vi "Finish.vi"   [LabVIEW 2013]
doc: "This VI is called just before exiting. It is expected to close I/O refnum, save collected data, etc."
uses:
  <vilib>/Rock Robotics/WPI/Joystick/WPI_JoystickGetSetRefNum.vi
types:
  T1 = typedef "WPI_MotorControlDeviceRef.ctl" = cluster{"DeviceStatus":errorcluster, "Type":enum16{"PWM", "CAN"}, "PWM":cluster{"Digital Module":T2, "PWM Channel":T3, "DeadBand":T4}, "CAN":cluster{"Device Number":u8, "Control Mode":T5, "Semaphore":T6, "Max Vout":dbl}, "Invert":bool, "TransformRef":T7, "InvTransformRef":T7}
  T2 = typedef "FPGA_TypedefDigitalModule.ctl" = enum16{"Digital Module 1", "Digital Module 2"}
  T3 = typedef "FPGA_DIOPWMChannel.ctl" = enum8{"PWM 1", "PWM 2", "PWM 3", "PWM 4", "PWM 5", "PWM 6", "PWM 7", "PWM 8", "PWM 9", "PWM 10", "Invalid"}
  T4 = typedef "WPI_PWMDeadband.ctl" = cluster{"Name":string, "maxPositivePwm":i32, "minPositivePwm":i32, "centerPwm":i32, "maxNegativePwm":i32, "minNegativePwm":i32, "angularRange":u16}
  T5 = typedef "WPI_CANJaguar_ControlMode.ctl" = enum8{"Percent VBus", "Current", "Speed", "Position", "Voltage"}
  T6 = typedef "Semaphore RefNum" = refnum<k1>
  T7 = typedef "WPI_PWMTransform_ConPane.ctl" = refnum<vi>
  T8 = typedef "WPI_JoystickDevRef.ctl" = cluster{"Device":T9}
  T9 = typedef "WPI_JoystickDeviceEnum.ctl" = enum16{"USB 1", "USB 2", "USB 3", "USB 4", "Kinect 1", "Kinect 2"}
  T10 = typedef "WPI_CounterDevRef.ctl" = cluster{"DevStatus":errorcluster, "CntIndex":T11}
  T11 = typedef "FPGA_CounterCtrSystemIndex.ctl" = enum8{"Ctr 0", "Ctr 1", "Ctr 2", "Ctr 3", "Ctr 4", "Ctr 5", "Ctr 6", "Ctr 7", "Invalid"}
  T12 = typedef "WPI_SolenoidDevRef.ctl" = cluster{"DevStatus":errorcluster, "Solenoid Module":T13, "Forward Solenoid Channel":T14, "Reverse Solenoid Channel":T14}
  T13 = typedef "FPGA_TypedefSolenoidModule.ctl" = enum16{"Solenoid Module 1", "Solenoid Module 2"}
  T14 = typedef "WPI_SolenoidChannel.ctl" = enum8{"Solenoid 1", "Solenoid 2", "Solenoid 3", "Solenoid 4", "Solenoid 5", "Solenoid 6", "Solenoid 7", "Solenoid 8", "Invalid"}
  T15 = typedef "WPI_AnalogChannelDevRef.ctl" = cluster{"DevStatus":errorcluster, "Analog Module":T16, "Analog Channel":T17}
  T16 = typedef "FPGA_TypedefAnalogModule.ctl" = enum16{"Analog Module 1", "Analog Module 2"}
  T17 = typedef "FPGA_AIChannel.ctl" = enum8{"AI 1", "AI 2", "AI 3", "AI 4", "AI 5", "AI 6", "AI 7", "AI 8", "Invalid"}
  T18 = typedef "WPI_DigitalInputDevRef.ctl" = cluster{"DevStatus":errorcluster, "DIO Channel":T19, "Digital Module":T2}
  T19 = typedef "FPGA_DIOChannel.ctl" = enum8{"DIO 1", "DIO 2", "DIO 3", "DIO 4", "DIO 5", "DIO 6", "DIO 7", "DIO 8", "DIO 9", "DIO 10", "DIO 11", "DIO 12", "DIO 13", "DIO 14", "Invalid"}
  T20 = typedef "WPI_GyroDevRef.ctl" = cluster{"DevStatus":errorcluster, "Analog Module":T16, "Analog Channel":T17, "Offset":dbl, "Gain (VoltsPerDegree/Second)":dbl}
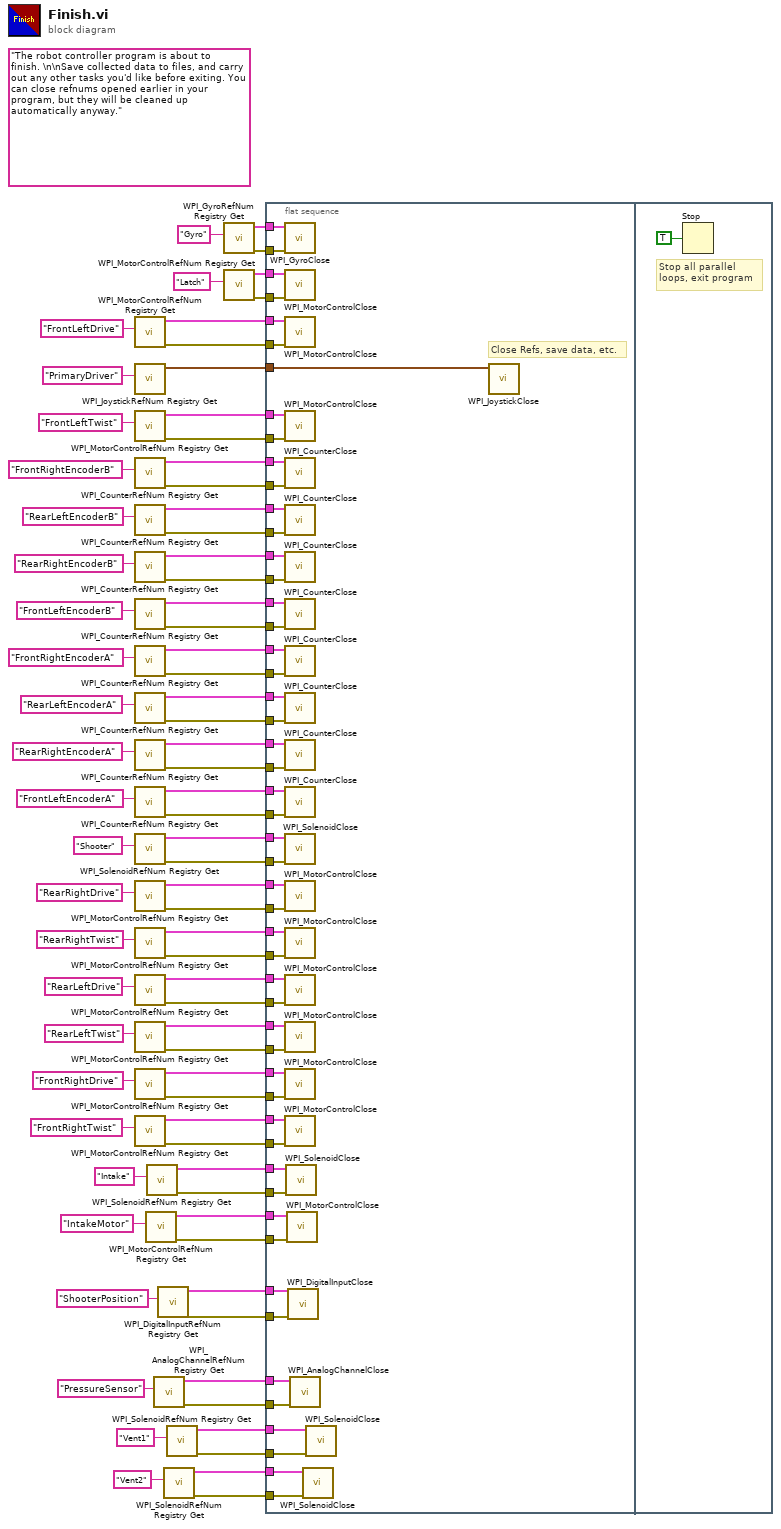
[diagram p0: block diagram]
diagram:
  (unwired) "The robot controller program is about to finish. \n\nSave collected data to files, and carry out any other tasks you'd like before exiting. You can close refnums opened earlier in your program, but they will be cleaned up automatically anyway."
  n1 = call <vilib>:"WPI_MotorControlRefNum Registry Get.vi"("refnum name"="FrontLeftDrive") -> ("error out"=w70:errorcluster, "MotorControlDevRef"=w71:T1)  [unwired: 9 in]
  n2 = call <vilib>:"WPI_JoystickRefNum Registry Get.vi"("refnum name"="PrimaryDriver") -> ("JoystickDevRef"=w77:T8)  [unwired: 9 in, 1 out]
  n3 = call <vilib>:"WPI_MotorControlRefNum Registry Get.vi"("refnum name"="FrontLeftTwist") -> ("error out"=w74:errorcluster, "MotorControlDevRef"=w75:T1)  [unwired: 9 in]
  n4 = call <vilib>:"WPI_CounterRefNum Registry Get.vi"("refnum name"="FrontRightEncoderB") -> ("error out"=w30:errorcluster, "CounterDevRef"=w29:T10)  [unwired: 9 in]
  n5 = call <vilib>:"WPI_CounterRefNum Registry Get.vi"("refnum name"="RearLeftEncoderB") -> ("error out"=w31:errorcluster, "CounterDevRef"=w28:T10)  [unwired: 9 in]
  n6 = call <vilib>:"WPI_CounterRefNum Registry Get.vi"("refnum name"="RearRightEncoderB") -> ("error out"=w32:errorcluster, "CounterDevRef"=w27:T10)  [unwired: 9 in]
  n7 = call <vilib>:"WPI_CounterRefNum Registry Get.vi"("refnum name"="FrontLeftEncoderB") -> ("error out"=w33:errorcluster, "CounterDevRef"=w26:T10)  [unwired: 9 in]
  n8 = call <vilib>:"WPI_CounterRefNum Registry Get.vi"("refnum name"="FrontRightEncoderA") -> ("error out"=w37:errorcluster, "CounterDevRef"=w38:T10)  [unwired: 9 in]
  n9 = call <vilib>:"WPI_CounterRefNum Registry Get.vi"("refnum name"="RearLeftEncoderA") -> ("error out"=w36:errorcluster, "CounterDevRef"=w39:T10)  [unwired: 9 in]
  n10 = call <vilib>:"WPI_CounterRefNum Registry Get.vi"("refnum name"="RearRightEncoderA") -> ("error out"=w35:errorcluster, "CounterDevRef"=w40:T10)  [unwired: 9 in]
  n11 = call <vilib>:"WPI_CounterRefNum Registry Get.vi"("refnum name"="FrontLeftEncoderA") -> ("error out"=w34:errorcluster, "CounterDevRef"=w41:T10)  [unwired: 9 in]
  n12 = call <vilib>:"WPI_SolenoidRefNum Registry Get.vi"("refnum name"="Shooter") -> ("error out"=w47:errorcluster, "SolenoidDevRef"=w48:T12)  [unwired: 9 in]
  n13 = call <vilib>:"WPI_MotorControlRefNum Registry Get.vi"("refnum name"="RearRightDrive") -> ("error out"=w57:errorcluster, "MotorControlDevRef"=w56:T1)  [unwired: 9 in]
  n14 = call <vilib>:"WPI_MotorControlRefNum Registry Get.vi"("refnum name"="RearRightTwist") -> ("error out"=w55:errorcluster, "MotorControlDevRef"=w54:T1)  [unwired: 9 in]
  n15 = call <vilib>:"WPI_MotorControlRefNum Registry Get.vi"("refnum name"="RearLeftDrive") -> ("error out"=w58:errorcluster, "MotorControlDevRef"=w59:T1)  [unwired: 9 in]
  n16 = call <vilib>:"WPI_MotorControlRefNum Registry Get.vi"("refnum name"="RearLeftTwist") -> ("error out"=w60:errorcluster, "MotorControlDevRef"=w61:T1)  [unwired: 9 in]
  n17 = call <vilib>:"WPI_MotorControlRefNum Registry Get.vi"("refnum name"="FrontRightDrive") -> ("error out"=w64:errorcluster, "MotorControlDevRef"=w65:T1)  [unwired: 9 in]
  n18 = call <vilib>:"WPI_MotorControlRefNum Registry Get.vi"("refnum name"="FrontRightTwist") -> ("error out"=w66:errorcluster, "MotorControlDevRef"=w67:T1)  [unwired: 9 in]
  n19 = call <vilib>:"WPI_MotorControlRefNum Registry Get.vi"("refnum name"="IntakeMotor") -> ("error out"=w18:errorcluster, "MotorControlDevRef"=w17:T1)  [unwired: 9 in]
  n20 = call <vilib>:"WPI_SolenoidRefNum Registry Get.vi"("refnum name"="Intake") -> ("error out"=w14:errorcluster, "SolenoidDevRef"=w13:T12)  [unwired: 9 in]
  n21 = call <vilib>:"WPI_AnalogChannelRefNum Registry Get.vi"("refnum name"="PressureSensor") -> ("error out"=w8:errorcluster, "AIDeviceRef"=w9:T15)  [unwired: 9 in]
  n22 = call <vilib>:"WPI_DigitalInputRefNum Registry Get.vi"("refnum name"="ShooterPosition") -> ("error out"=w11:errorcluster, "DigitalInputDevRef"=w12:T18)  [unwired: 9 in]
  n23 = call <vilib>:"WPI_SolenoidRefNum Registry Get.vi"("refnum name"="Vent2") -> ("error out"=w2:errorcluster, "SolenoidDevRef"=w1:T12)  [unwired: 9 in]
  n24 = call <vilib>:"WPI_SolenoidRefNum Registry Get.vi"("refnum name"="Vent1") -> ("error out"=w5:errorcluster, "SolenoidDevRef"=w6:T12)  [unwired: 9 in]
  n25 = call <vilib>:"WPI_GyroRefNum Registry Get.vi"("refnum name"="Gyro") -> ("error out"=w20:errorcluster, "GyroDevRef"=w21:T20)  [unwired: 9 in]
  n26 = call <vilib>:"WPI_MotorControlRefNum Registry Get.vi"("refnum name"="Latch") -> ("error out"=w49:errorcluster, "MotorControlDevRef"=w50:T1)  [unwired: 9 in]
  n27 = flat-sequence {
    tunnel: w77 -> [w128]
    tunnel: w75 -> [w127]
    tunnel: w74 -> [w126]
    tunnel: w71 -> [w124]
    tunnel: w70 -> [w125]
    tunnel: w67 -> [w123]
    tunnel: w66 -> [w122]
    tunnel: w65 -> [w121]
    tunnel: w64 -> [w120]
    tunnel: w61 -> [w119]
    tunnel: w60 -> [w118]
    tunnel: w59 -> [w117]
    tunnel: w58 -> [w116]
    tunnel: w54 -> [w112]
    tunnel: w55 -> [w113]
    tunnel: w56 -> [w114]
    tunnel: w57 -> [w115]
    tunnel: w50 -> [w111]
    tunnel: w49 -> [w110]
    tunnel: w48 -> [w109]
    tunnel: w47 -> [w108]
    tunnel: w41 -> [w107]
    tunnel: w40 -> [w106]
    tunnel: w39 -> [w105]
    tunnel: w38 -> [w104]
    tunnel: w37 -> [w103]
    tunnel: w36 -> [w102]
    tunnel: w35 -> [w101]
    tunnel: w34 -> [w100]
    tunnel: w26 -> [w92]
    tunnel: w27 -> [w93]
    tunnel: w28 -> [w94]
    tunnel: w29 -> [w95]
    tunnel: w30 -> [w96]
    tunnel: w31 -> [w97]
    tunnel: w32 -> [w98]
    tunnel: w33 -> [w99]
    tunnel: w21 -> [w91]
    tunnel: w20 -> [w90]
    tunnel: w17 -> [w88]
    tunnel: w18 -> [w89]
    tunnel: w13 -> [w86]
    tunnel: w14 -> [w87]
    tunnel: w12 -> [w85]
    tunnel: w11 -> [w84]
    tunnel: w9 -> [w83]
    tunnel: w8 -> [w82]
    tunnel: w6 -> [w81]
    tunnel: w5 -> [w80]
    tunnel: w1 -> [w78]
    tunnel: w2 -> [w79]
    frame #0 {
      # "Close Refs, save data, etc."
      n28 = call <vilib>:"WPI_GyroClose.vi"("error in (no error)"=w90, "GyroDevRef"=w91) -> ()  [unwired: 9 in, 1 out]
      n29 = call <vilib>:"WPI_MotorControlClose.vi"("error in (no error)"=w110, "MotorControlDevRef"=w111) -> ()  [unwired: 9 in, 1 out]
      n30 = call <vilib>:"WPI_MotorControlClose.vi"("error in (no error)"=w125, "MotorControlDevRef"=w124) -> ()  [unwired: 9 in, 1 out]
      n31 = call <vilib>:"WPI_MotorControlClose.vi"("error in (no error)"=w126, "MotorControlDevRef"=w127) -> ()  [unwired: 9 in, 1 out]
      n32 = call <vilib>:"WPI_CounterClose.vi"("error in (no error)"=w96, "CounterDevRef"=w95) -> ()  [unwired: 9 in, 1 out]
      n33 = call <vilib>:"WPI_CounterClose.vi"("error in (no error)"=w97, "CounterDevRef"=w94) -> ()  [unwired: 9 in, 1 out]
      n34 = call <vilib>:"WPI_CounterClose.vi"("error in (no error)"=w98, "CounterDevRef"=w93) -> ()  [unwired: 9 in, 1 out]
      n35 = call <vilib>:"WPI_CounterClose.vi"("error in (no error)"=w99, "CounterDevRef"=w92) -> ()  [unwired: 9 in, 1 out]
      n36 = call <vilib>:"WPI_CounterClose.vi"("error in (no error)"=w103, "CounterDevRef"=w104) -> ()  [unwired: 9 in, 1 out]
      n37 = call <vilib>:"WPI_CounterClose.vi"("error in (no error)"=w102, "CounterDevRef"=w105) -> ()  [unwired: 9 in, 1 out]
      n38 = call <vilib>:"WPI_CounterClose.vi"("error in (no error)"=w101, "CounterDevRef"=w106) -> ()  [unwired: 9 in, 1 out]
      n39 = call <vilib>:"WPI_CounterClose.vi"("error in (no error)"=w100, "CounterDevRef"=w107) -> ()  [unwired: 9 in, 1 out]
      n40 = call <vilib>:"WPI_SolenoidClose.vi"("error in (no error)"=w108, "SolenoidDevRef"=w109) -> ()  [unwired: 9 in, 1 out]
      n41 = call <vilib>:"WPI_MotorControlClose.vi"("error in (no error)"=w115, "MotorControlDevRef"=w114) -> ()  [unwired: 9 in, 1 out]
      n42 = call <vilib>:"WPI_MotorControlClose.vi"("error in (no error)"=w113, "MotorControlDevRef"=w112) -> ()  [unwired: 9 in, 1 out]
      n43 = call <vilib>:"WPI_MotorControlClose.vi"("error in (no error)"=w116, "MotorControlDevRef"=w117) -> ()  [unwired: 9 in, 1 out]
      n44 = call <vilib>:"WPI_MotorControlClose.vi"("error in (no error)"=w118, "MotorControlDevRef"=w119) -> ()  [unwired: 9 in, 1 out]
      n45 = call <vilib>:"WPI_MotorControlClose.vi"("error in (no error)"=w120, "MotorControlDevRef"=w121) -> ()  [unwired: 9 in, 1 out]
      n46 = call <vilib>:"WPI_MotorControlClose.vi"("error in (no error)"=w122, "MotorControlDevRef"=w123) -> ()  [unwired: 9 in, 1 out]
      n47 = call <vilib>:"WPI_SolenoidClose.vi"("error in (no error)"=w87, "SolenoidDevRef"=w86) -> ()  [unwired: 9 in, 1 out]
      n48 = call <vilib>:"WPI_MotorControlClose.vi"("error in (no error)"=w89, "MotorControlDevRef"=w88) -> ()  [unwired: 9 in, 1 out]
      n49 = call <vilib>:"WPI_DigitalInputClose.vi"("error in (no error)"=w84, "DigitalInputDevRef"=w85) -> ()  [unwired: 9 in, 1 out]
      n50 = call <vilib>:"WPI_AnalogChannelClose.vi"("error in (no error)"=w82, "AIDeviceRef"=w83) -> ()  [unwired: 9 in, 1 out]
      n51 = call <vilib>:"WPI_SolenoidClose.vi"("error in (no error)"=w79, "SolenoidDevRef"=w78) -> ()  [unwired: 9 in, 1 out]
      n52 = call <vilib>:"WPI_SolenoidClose.vi"("error in (no error)"=w80, "SolenoidDevRef"=w81) -> ()  [unwired: 9 in, 1 out]
      n53 = call <vilib>:"WPI_JoystickClose.vi"("JoystickDevRef"=w128) -> ()  [unwired: 11 in]
    }
    frame #1 {
      # "Stop all parallel\nloops, exit program"
      n54 = Stop(stop? (T)=TRUE ("Quit")) -> ()
    }
  }
